vi "Format for Tree Control.vi"(8 "Error In":errorcluster, 9 "Class Name":string, 10 "Attr Name":string, 11 "Tree Data":refnum<class "Tree Data.lvclass">) -> (0 "Error Out":errorcluster, 3 "Child Text":string[](array[string]))   [LabVIEW 2020, in "NI_VIAnCFGDataStructure.lvlib" / "Tree Data.lvclass"]
doc: "This method formats the string data for visualization in Tree Control. For most use cases it can stay default but if you want to have special strings for your own type, override it in child classes of Tree Data."
uses:
  <vilib>/addons/analyzer/VIAnCFGDataStructure/Tree Data/Tree Data.lvclass
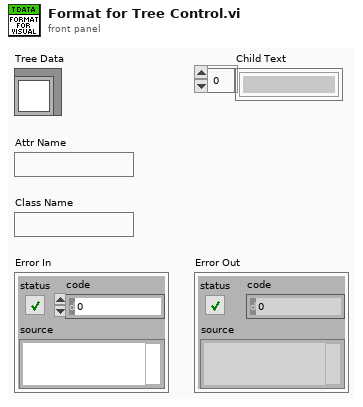
[diagram p1: front panel]
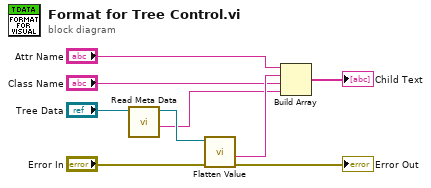
[diagram p0: block diagram]
diagram:
  n1 = call <vilib>:"Read Meta Data.vi"("Tree Data In"="Tree Data") -> ("Meta Data"=w4:string, "Tree Data Out"=w9:refnum<class "Tree Data.lvclass">)  [unwired: 9 in]
  n2 = call-dynamic "Flatten Value.vi"("Error In"="Error In", "Tree Data In"=w9) -> ("Error Out"=→"Error Out":errorcluster, "Value"=w6:string)  [unwired: 7 in, 1 out]
  n3 = Build Array("Attr Name", w6, "Class Name", w4) -> (→"Child Text":string[])
